vi "Convert Image Coordinates to Angles.vi"(9 "Focal length in pixels":dbl, 10 "Corner":cluster{"X":dbl, "Y":dbl}, 11 "Camera Resolution":T1={"Camera Resolution W (pixels)"=800.0, "Camera Resolution H (pixels)"=600.0}) -> (2 "Thata Y":dbl, 3 "Thata Z":dbl)   [LabVIEW 2023]
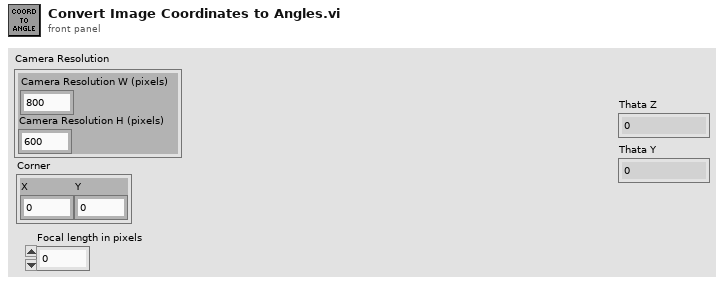
[diagram p1: front panel]
types:
  T1 = cluster{"Camera Resolution W (pixels)":dbl, "Camera Resolution H (pixels)":dbl}
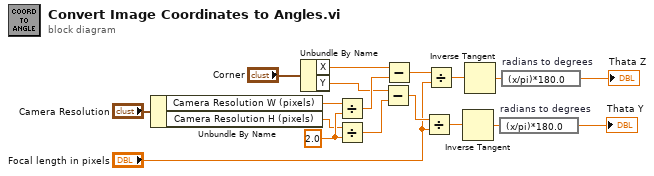
[diagram p0: block diagram]
diagram:
  w18 = 2.0 ("y")
  n1 = Unbundle By Name("Camera Resolution") -> ("Camera Resolution W (pixels)"=w16:dbl, "Camera Resolution H (pixels)"=w15:dbl)
  n2 = Unbundle By Name("Corner") -> ("X"=w13:dbl, "Y"=w11:dbl)
  n3 = Divide(x=w16, y=w18) -> (x/y=w12:dbl)
  n4 = Divide(x=w15, y=w18) -> (x/y=w10:dbl)
  n5 = Subtract(x=w11, y=w10) -> (x-y=w2:dbl)
  n6 = Subtract(x=w13, y=w12) -> (x-y=w9:dbl)
  n7 = Divide(x=w2, y="Focal length in pixels") -> (x/y=w3:dbl)
  n8 = Divide(x=w9, y="Focal length in pixels") -> (x/y=w8:dbl)
  n9 = Inverse Tangent(1:w3) -> (0:w4:dbl)
  n10 = Inverse Tangent(1:w8) -> (0:w7:dbl)
  n11 = expression code="(x/pi)*180.0" "radians to degrees"(w4) -> (→"Thata Y":dbl)
  n12 = expression code="(x/pi)*180.0" "radians to degrees"(w7) -> (→"Thata Z":dbl)
